vi "Write High Limit.vi"(8 "error in":errorcluster, 10 "high limit":variant, 11 "Has Control Limits in":refnum<class "Has Control Limits.lvclass">) -> (0 "error out":errorcluster, 3 "Has Control Limits out":refnum<class "Has Control Limits.lvclass">)   [LabVIEW 2020, in "PV Access.lvlib" / "PV Data.lvlib" / "Has Control Limits.lvclass"]
uses:
  Has Control Limits.lvclass
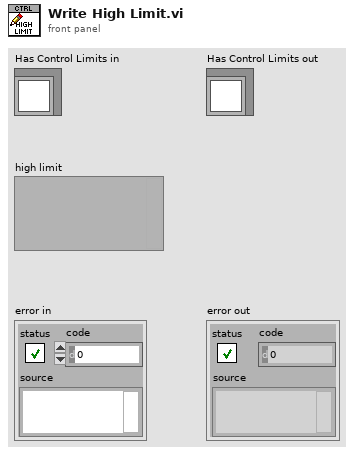
[diagram p1: front panel]
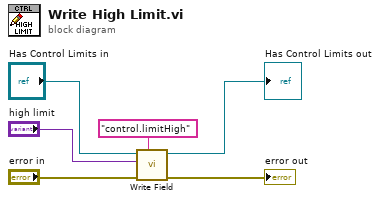
[diagram p0: block diagram]
diagram:
  n1 = call-dynamic "Write Field.vi"("field"="control.limitHigh" ("element name"), "error in (no error)"="error in", "value"="high limit", "Base Interface in"="Has Control Limits in") -> ("error out"=→"error out":errorcluster, "Base Interface out"=→"Has Control Limits out":refnum<class "Has Control Limits.lvclass">)  [unwired: 6 in]
